vi "未命名 8.vi"(8 "错误输入（无错误）":errorcluster, 10 "单元格":T2, 11 "引用":refnum<vi>) -> (0 "错误输出":errorcluster, 2 "单元格位置":T1, 3 "引用输出":refnum<vi>)   [LabVIEW 2014, in "表格.lvlib"]
uses:
  <vilib>/Utility/miscctls.llb/LVRowAndColumnTypeDef.ctl
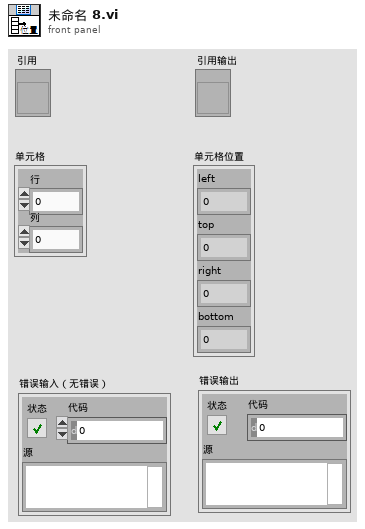
[diagram p1: front panel]
types:
  T1 = cluster{"left":i16, "top":i16, "right":i16, "bottom":i16}
  T2 = typedef "LVRowAndColumnTypeDef.ctl" = cluster{"Row":i32, "Column":i32}
  T3 = typedef "LVPositionTypeDef.ctl" = cluster{"Left":i32, "Top":i32}
  T4 = typedef "LVBoundsTypeDef.ctl" = cluster{"Width":u32, "Height":u32}
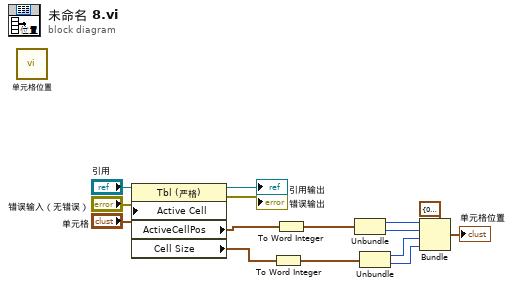
[diagram p0: block diagram]
diagram:
  n1 = call "单元格位置.vi"() -> ()  [unwired: 9 in, 3 out]
  n2 = property on="Property Node" class="Tbl (严格)"(reference="引用", error in="错误输入（无错误）", "Active Cell"="单元格") -> (reference out=→"引用输出":refnum<vi>, error out=→"错误输出":errorcluster, "ActiveCellPos"=w10:T3, "Cell Size"=w9:T4)
  n3 = To Word Integer(number=w9) -> (16bit integer=w7:cluster{"Width":i16, "Height":i16})
  n4 = To Word Integer(number=w10) -> (16bit integer=w15:cluster{"Left":i16, "Top":i16})
  n5 = Unbundle(w15) -> ("Left"=w11:i16, "Top"=w12:i16)
  n6 = Unbundle(w7) -> ("Width"=w13:i16, "Height"=w14:i16)
  n7 = Bundle(cluster=T1 {"left"=0, "top"=0, "right"=0, "bottom"=0} ("Cell Rect Out"), "left"=w11, "top"=w12, "right"=w13, "bottom"=w14) -> (→"单元格位置":T1)
